vi "Day 17 Rock Formation.vi"(0 "Chamber":u32[][](array[colorbox])) -> (1 "Rock Formation":string, 2 "Rock Formation with Shapes":string)   [LabVIEW 2020, in "AoC 2022.lvlib"]
uses:
  AoC 2022.lvlib
  Day 17 - Pyroclastic Flow/private/Pyroclastic Rock Shape.ctl
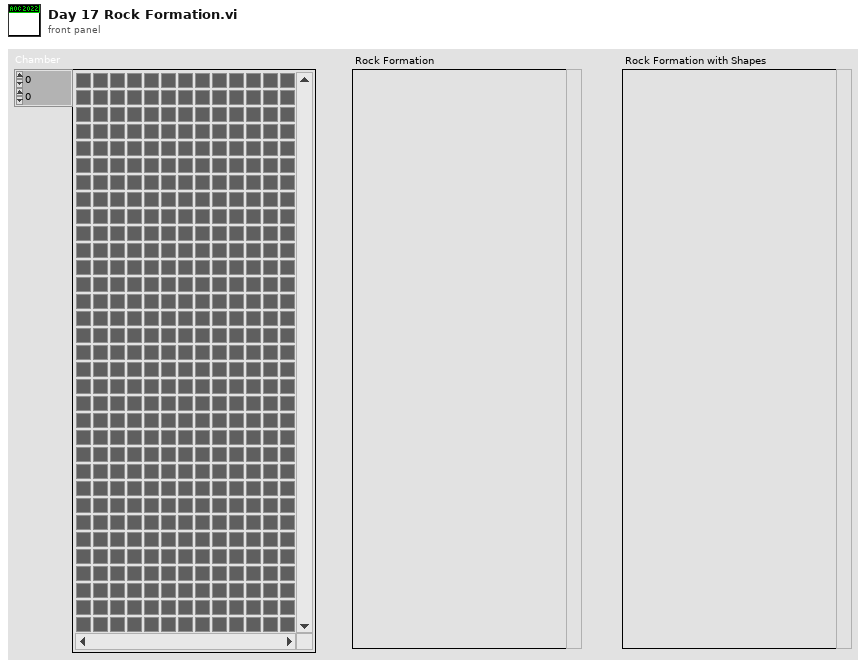
[diagram p1: front panel]
types:
  T1 = typedef "AoC 2022.lvlib/Pyroclastic Rock Shape.ctl" = enum16{"_", "+", "_|", "|", "."}
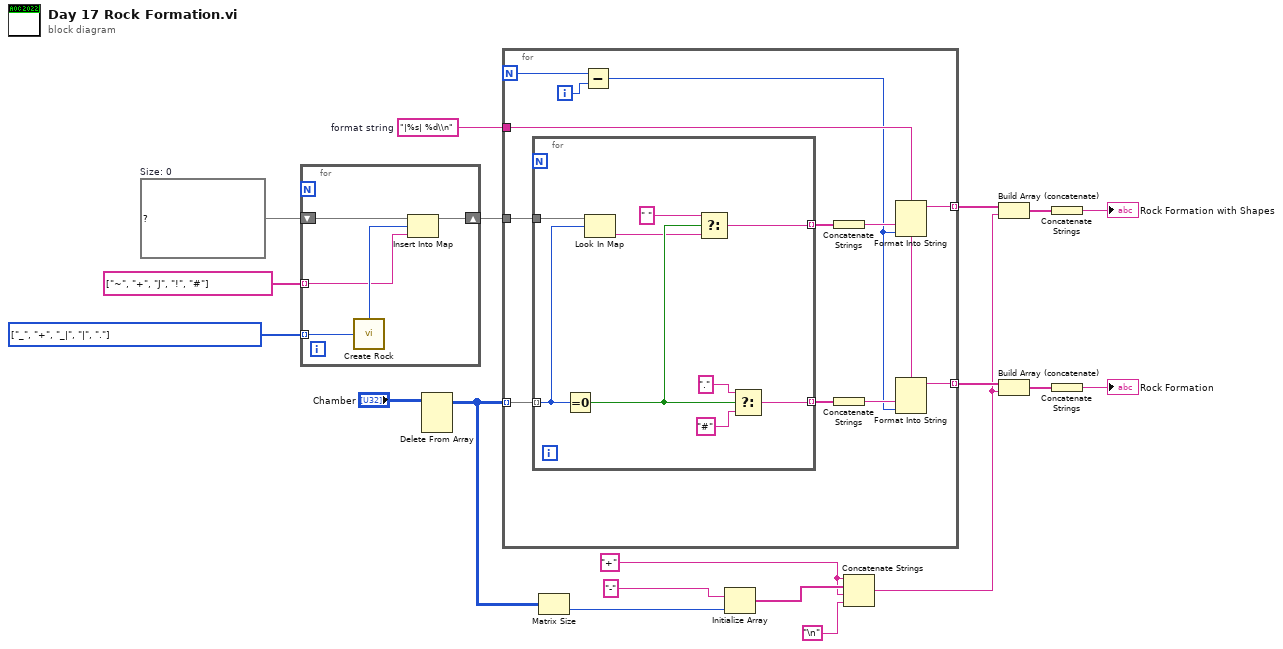
[diagram p0: block diagram]
diagram:
  w5 = "|%s| %d\\n"  # format string
  w7 = T1[] [enum."_", enum."+", enum."_|", enum."|", enum."."] items=["_", "+", "_|", "|", "."]
  w9 = map{u32, string} {}  # Size: 0
  w13 = "+"
  n1 = for {
    tunnel: w7 -> [w24] mode=indexing
    shift-right: [w21] -> w6
    shift-left: w9 -> [w23]
    tunnel: string[] ["~", "+", "J", "!", "#"] -> [w20] mode=indexing
    n2 = call "Create Rock.vi"("Pyroclastic Rock Shape"=w24) -> ("Rock Color"=w22:u32)  [unwired: 1 out]
    n3 = Insert Into Map(map in=w23, key=w22, value=w20) -> (map out=w21:map{u32, string})  [unwired: 2 out]
  }
  n4 = Delete From Array(array="Chamber") -> (array with subset deleted=w10:u32[][])  [unwired: 3 in, 1 out]
  n5 = for {
    N -> [w34]
    tunnel: w10 -> [w36] mode=indexing
    tunnel: [w30] -> w19 mode=indexing
    tunnel: w6 -> [w35]
    tunnel: w5 -> [w28]
    tunnel: [w25] -> w4 mode=indexing
    i -> [w33]
    n6 = for {
      tunnel: w36 -> [w42] mode=indexing
      tunnel: [w38] -> w32 mode=indexing
      tunnel: w35 -> [w43]
      tunnel: [w37] -> w29 mode=indexing
      n7 = Equal To 0?(x=w42) -> (x = 0?=w40:bool)
      n8 = Look In Map(map=w43, key=w42) -> (value=w39:string)  [unwired: 1 in, 1 out]
      n9 = Select(t=" ", s=w40, f=w39) -> (s? t:f=w37:string)
      n10 = Select(t=".", s=w40, f="#") -> (s? t:f=w38:string)
    }
    n11 = Subtract(x=w34, y=w33) -> (x-y=w26:i32)
    n12 = Concatenate Strings(w29) -> (w27:string)
    n13 = Concatenate Strings(w32) -> (w31:string)
    n14 = Format Into String(format string=w28, w27, w26) -> (resulting string=w25:string)  [unwired: 2 in, 1 out]
    n15 = Format Into String(format string=w28, w31, w26) -> (resulting string=w30:string)  [unwired: 2 in, 1 out]
  }
  n16 = Matrix Size(0:w10) -> (2:w15:i32)  [unwired: 1 out]
  n17 = Initialize Array("-", w15) -> (w14:string[])
  n18 = Concatenate Strings(w13, w14, w13, "\n") -> (w3:string)
  n19 = Build Array (concatenate)(w4, w3) -> (w1:string[])
  n20 = Build Array (concatenate)(w19, w3) -> (w11:string[])
  n21 = Concatenate Strings(w1) -> (→"Rock Formation with Shapes":string)
  n22 = Concatenate Strings(w11) -> (→"Rock Formation":string)
